vi "框图整理.vi"() -> ()   [LabVIEW 2018]
uses:
  <vilib>/Utility/miscctls.llb/LVPositionTypeDef.ctl
panel:
  in  "不包含信号":string[](array[string])
  in  "不包含字符串":string[](array[string])
  in  "包含字符串":string[](array[string])
  in  "位置":T1
  in  "修改":bool
  out "数组":string[](array[string])
  in  "VI路径":path
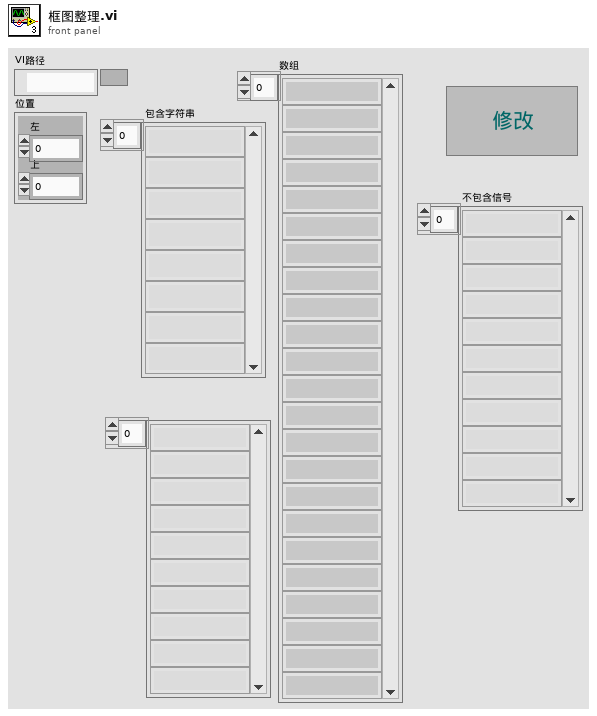
[diagram p1: front panel]
types:
  T1 = typedef "LVPositionTypeDef.ctl" = cluster{"Left":i32, "Top":i32}
  T2 = typedef "LVBoundsTypeDef.ctl" = cluster{"Width":u32, "Height":u32}
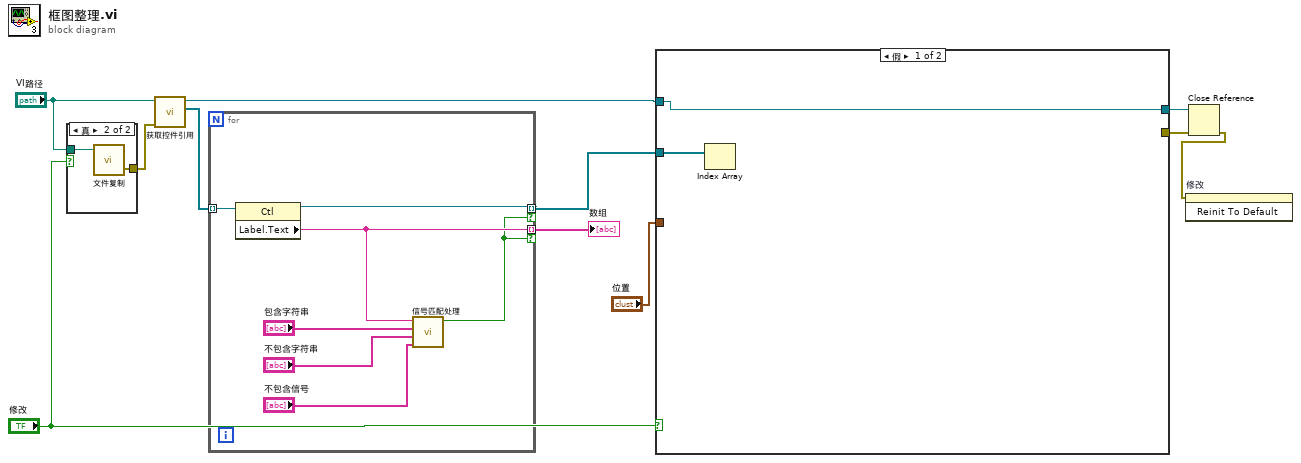
[diagram p0: block diagram]
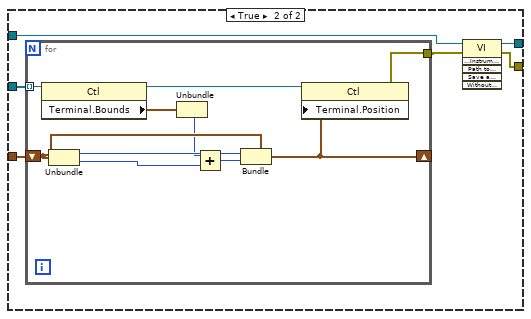
[diagram p3: hidden frame]
diagram:
  n1 = case shown="真" "修改" {
    tunnel: "VI路径" -> [_ w13]
    tunnel: [_ w12] -> w1
    frame False {
    }
    frame True {
      n2 = call "文件复制.vi"("VI路径"=w13) -> ("error out"=w12:errorcluster)  [unwired: 4 in]
    }
  }
  n3 = call "获取控件引用.vi"("错误输入（无错误）"=w1, "VI路径"="VI路径") -> ("ContrlRefArray"=w7:refnum<vi>[], "VIRef"=w10:refnum<vi>)  [unwired: 6 in, 1 out]
  n4 = for {
    tunnel: w7 -> [w20] mode=indexing
    tunnel: [w19] -> w6 mode=indexing if=w17
    tunnel: [w18] -> w5 mode=indexing if=w17
    n5 = property class="Ctl"(reference=w20) -> (reference out=w19:refnum<vi>, "Label.Text"=w18:string)  [unwired: 1 in, 1 out]
    n6 = call "信号匹配处理.vi"("不包含信号"="不包含信号", "不包含字符串"="不包含字符串", "包含字符串"="包含字符串", "输入字符串"=w18) -> ("匹配"=w17:bool)  [unwired: 7 in]
  }
  "数组" <- w5
  n7 = case shown="假" "修改" {
    tunnel: "位置" -> [_ w28]
    tunnel: w10 -> [w22 w27]
    tunnel: [w22 w26] -> w9
    tunnel: [_ w25] -> w8
    tunnel: w6 -> [w21 w24]
    frame False {
      n8 = Index Array(array=w21) -> ()  [unwired: 1 in, 1 out]
    }
    frame True {
      n9 = for {
        tunnel: w24 -> [w38] mode=indexing
        shift-right: [w30] -> _
        shift-left: w28 -> [w37]
        tunnel: [w29] -> w23
        n10 = property class="Ctl"(reference=w38) -> (reference out=w35:refnum<vi>, "Terminal.Bounds"=w34:T2)  [unwired: 1 in, 1 out]
        n11 = Unbundle(w37) -> ("Left"=w36:i32, "Top"=w31:i32)
        n12 = Unbundle(w34) -> ("Height"=w32:u32)  [unwired: 1 out]
        n13 = Add(x=w32, y=w31) -> (x+y=w33:u32)
        n14 = Bundle(cluster=w37, "Left"=w36, "Top"=w33) -> (w30:T1)
        n15 = property class="Ctl"(reference=w35, "Terminal.Position"=w30) -> (error out=w29:errorcluster)  [unwired: 1 in, 1 out]
      }
      n16 = invoke class="VI" method="Save.Instrument"(reference=w27, error in=w23) -> (reference out=w26:refnum<vi>, error out=w25:errorcluster)  [unwired: 4 in, 4 out]
    }
  }
  n17 = Close Reference(reference=w9, error in (no error)=w8) -> (error out=w4:errorcluster)
  n18 = invoke on="修改" class="Bool (严格)" method="Reinit To Default"(error in=w4) -> ()  [unwired: 2 in, 3 out]
